vi "Setlist_services_response.vi"(8 "error in (no error)":errorcluster, 10 "Set_Val":T1, 11 "OneOfTemplate in":refnum<class "grpc_reflection_v1alpha_ServerReflectionResponse_message_response.lvclass">) -> (0 "error out":errorcluster, 3 "OneOfTemplate out":refnum<class "grpc_reflection_v1alpha_ServerReflectionResponse_message_response.lvclass">)   [LabVIEW 2019, in "reflection_client.lvlib" / "grpc_reflection_v1alpha_ServerReflectionResponse_message_response.lvclass"]
uses:
  grpc_reflection_v1alpha_ServerReflectionResponse_message_response.lvclass
  grpc_reflection_v1alpha_ListServiceResponse.ctl
  grpc_reflection_v1alpha_ServiceResponse.ctl
  grpc_reflection_v1alpha_ServerReflectionResponse_message_response.lvclass/grpc_reflection_v1alpha_ServerReflectionResponse_message_response.ctl
  reflection_client.lvlib
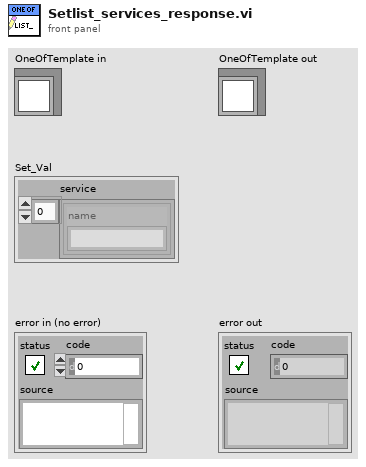
[diagram p1: front panel]
types:
  T1 = typedef "reflection_client.lvlib/grpc_reflection_v1alpha_ListServiceResponse.ctl" = cluster{"service":T2[]}
  T2 = typedef "reflection_client.lvlib/grpc_reflection_v1alpha_ServiceResponse.ctl" = cluster{"name":string}
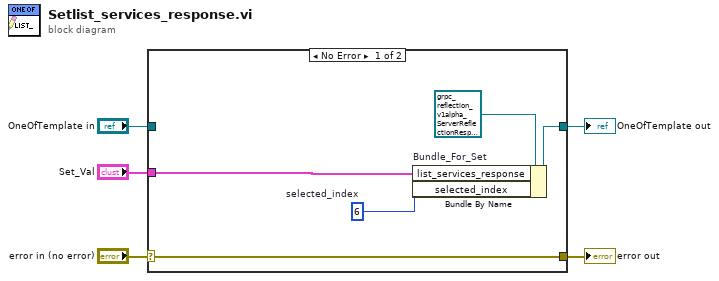
[diagram p0: block diagram]
diagram:
  n1 = case shown="No Error" "error in (no error)" {
    selector: "error in (no error)" -> [w10 w11]
    tunnel: [w10 w11] -> w4
    tunnel: [w9 w12] -> w2
    tunnel: "OneOfTemplate in" -> [_ w12]
    tunnel: "Set_Val" -> [w8 _]
    frame No Error {
      w7 = 6  # selected_index
      n2 = Bundle By Name "Bundle_For_Set"(cluster=refnum<class "grpc_reflection_v1alpha_ServerReflectionResponse_message_response.lvclass"> refnum ("OneOfTemplate in"), "list_services_response"=w8, "selected_index"=w7) -> (w9:refnum<class "grpc_reflection_v1alpha_ServerReflectionResponse_message_response.lvclass">)
    }
    frame Error {
    }
  }
  "error out" <- w4
  "OneOfTemplate out" <- w2
